vi "InitialTrayStatus.vi"(8 "error in (no error)":errorcluster, 11 "BarcodeScan in":refnum<class "BarcodeScan.lvclass">) -> (0 "error out":errorcluster, 3 "BarcodeScan out":refnum<class "BarcodeScan.lvclass">)   [LabVIEW 2019, in "BarcodeScan.lvclass"]
uses:
  BarcodeScan.lvclass
  FlowIOCtrl.lvclass
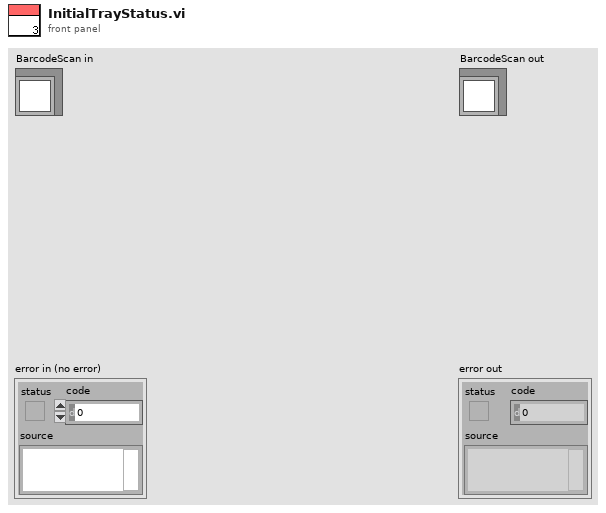
[diagram p1: front panel]
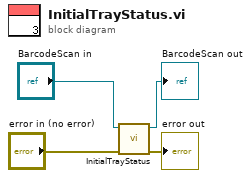
[diagram p0: block diagram]
diagram:
  n1 = call-parent "InitialTrayStatus.vi"("error in (no error)"="error in (no error)", "Station Action in"="BarcodeScan in") -> ("error out"=→"error out":errorcluster, "Station Action out"=→"BarcodeScan out":refnum<class "BarcodeScan.lvclass">)  [unwired: 8 in]
